vi "Task2.vi"() -> ()   [LabVIEW 2019]
uses:
  <vilib>/addons/Control Design/_Model Construction/Data Typedefs.llb/CD Variables.ctl
  <vilib>/addons/Control Design/_Model Construction/Model Creation.llb/Model Creation SubVI/cd_Create Symbolic Transfer Function Model.vi
  <vilib>/addons/Control Design/_Utility/Model Viewer.llb/Model Viewer SubVI/cd_Draw Transfer Function Equation (TF).vi
  <vilib>/addons/Control Design/_Model Construction/NI_LinSys_Model Creation.lvlib
  <vilib>/addons/Control Design/_Utility/NI_CD_Model Viewer.lvlib
  <vilib>/addons/Control Design/_Model Construction/NI_LinSys_Data Typedefs.lvlib
panel:
  out "Plant Equation 2":picture
  in  "Variables":T1 {"Value" format="%.2f"}
  in  "Symbolic Numerator":string[](array[string])
  in  "Symbolic Denominator":string[](array[string])
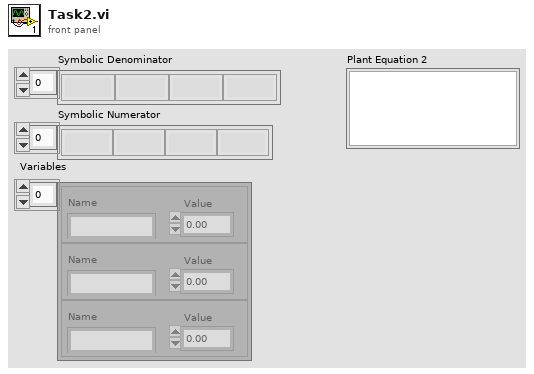
[diagram p1: front panel]
types:
  T1 = typedef "NI_LinSys_Data Typedefs.lvlib/CD Variables.ctl" = cluster{"Name":string, " Value":dbl}[]
  T2 = typedef "NI_LinSys_Model Typedefs.lvlib/CD Transfer Function Model (MIMO).ctl" = cluster{"properties":T3, "transfer function(s)":T4[][]}
  T3 = typedef "NI_LinSys_Model Typedefs.lvlib/CD General Elements.ctl" = cluster{"Model name":string, "Input names":string[], "Output names":string[], "Input Delays":dbl[], "Output Delays":dbl[], "Sampling Time":dbl, "Notes":string}
  T4 = typedef "NI_LinSys_Model Typedefs.lvlib/CD Transfer Function Model (SISO).ctl" = cluster{"Numerator":dbl[], "Denominator":dbl[], "delay":dbl}
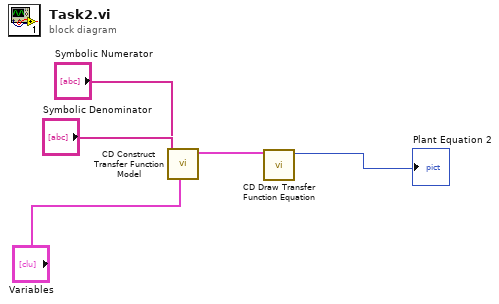
[diagram p0: block diagram]
diagram:
  n1 = call-poly <vilib>:"CD Construct Transfer Function Model.vi"("Variables"="Variables", "Symbolic Denominator"="Symbolic Denominator", "Symbolic Numerator"="Symbolic Numerator") -> ("Transfer Function Model"=w2:T2)  [unwired: 7 in, 1 out]
  n2 = call-poly <vilib>:"CD Draw Transfer Function Equation.vi"("Transfer Function Model"=w2) -> ("Equation"=→"Plant Equation 2":picture)  [unwired: 8 in, 2 out]
